vi "Image to File.vi"(7 "Control Ref Queue":T1, 8 "error in ( no error )":errorcluster, 9 "Path":path, 10 "Target":enum32{"File", "Clipboard"}(ring), 11 "File Type":enum32{"BMP", "EPS", "EMF", "PICT"}(ring)) -> (0 "error out":errorcluster)   [LabVIEW 2020, in "3D Plot.lvclass"]
uses:
  3D Plot.lvclass
  3DMathPlot Ctrl Act Queue.ctl
  3DMathPlot Ctrl Act Cluster.ctl
  3DMathPlot State Class.ctl
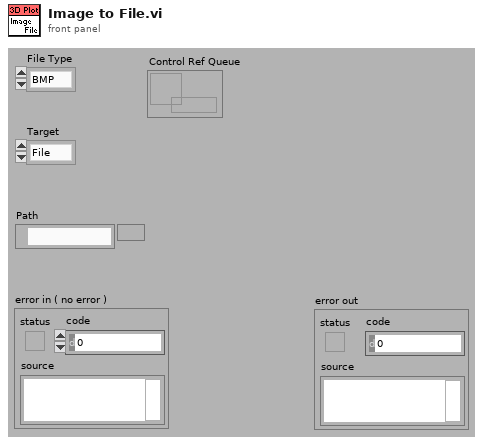
[diagram p1: front panel]
types:
  T1 = typedef "3DMathPlot Ctrl Act Queue.ctl" = refnum<queue>
  T2 = typedef "3DMathPlot Ctrl Act Cluster.ctl" = cluster{"3D Picture Control":refnum<vi>, "Render Window Refnum":refnum<vi>, "XY Graph":refnum<vi>, "Intensity Graph":refnum<vi>, "Color Legend Palette":refnum<vi>, "Projection Palette":refnum<vi>, "XControl  Ref":refnum<vi>, "Facade Ref":refnum<vi>, "Export Image Ref":refnum<vi>, "Clear Data Flag":bool, "Display State Change Class":T3}
  T3 = typedef "3DMathPlot State Class.ctl" = enum16{"Update All Objects (Undo)", "Update Light Object Only", "Update Axis Object Only", "Update Plot Object Only", "Update Cursor Object Only", "Update Axis Plot Cursor Objects", "No Update"}
  T4 = typedef "imagedata.ctl" = cluster{"image type":i32, "image depth":i32, "image":u8[], "mask":u8[], "colors":u32[], "Rectangle":cluster{"left":i16, "top":i16, "right":i16, "bottom":i16}}
  T5 = typedef "LVBoundsTypeDef.ctl" = cluster{"Width":u32, "Height":u32}
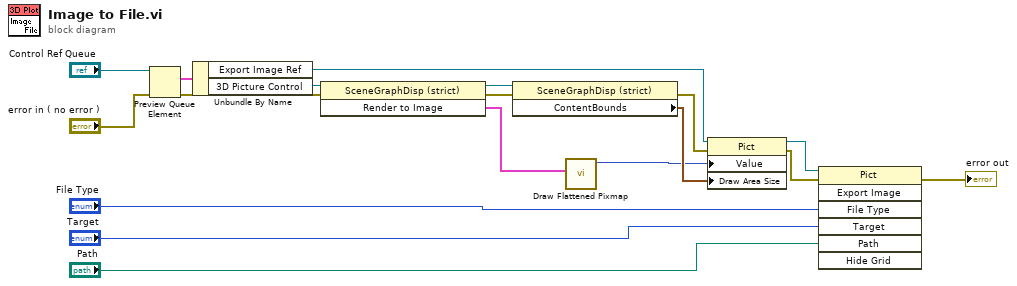
[diagram p0: block diagram]
diagram:
  n1 = Preview Queue Element(queue="Control Ref Queue", error in (no error)="error in ( no error )") -> (element=w3:T2, error out=w6:errorcluster)  [unwired: 3 out]
  n2 = Unbundle By Name(w3) -> ("Export Image Ref"=w1:refnum<vi>, "3D Picture Control"=w5:refnum<vi>)
  n3 = invoke on="Invoke Node" class="SceneGraphDisp (strict)" method="Render to Image"(reference=w5, error in=w6) -> (reference out=w9:refnum<vi>, error out=w11:errorcluster, "Get Image"=w7:T4)  [unwired: 1 in]
  n4 = property class="SceneGraphDisp (strict)"(reference=w9, error in=w11) -> (error out=w12:errorcluster, "ContentBounds"=w10:T5)  [unwired: 1 out]
  n5 = call "Draw Flattened Pixmap.vi"("image data"=w7) -> ("new picture"=w8:picture)  [unwired: 1 in, 7 out]
  n6 = property on="Property Node" class="Pict"(reference=w1, error in=w12, "Value"=w8, "Draw Area Size"=w10) -> (reference out=w2:refnum<vi>, error out=w4:errorcluster)
  n7 = invoke on="Invoke Node" class="Pict" method="Export Image"(reference=w2, error in=w4, "File Type"="File Type", "Target"="Target", "Path"="Path") -> (error out=→"error out":errorcluster)  [unwired: 2 in, 6 out]
